vi "CalculateStartupRMS.vi"(8 "error in (no error)":errorcluster, 9 "frequency":dbl, 10 "Motor":T1, 11 "current waveforms":waveform(dbl)[](array[waveform])) -> (0 "error out":errorcluster, 3 "Percent Full Load Amps [%FLA]":dbl)   [LabVIEW 2017, in "McsaAnalysisFunctions.lvlib"]
uses:
  <vilib>/addons/InsightCM/Utilities/Analysis/MCSA/McsaAnalysisFunctions.lvlib
  <vilib>/addons/InsightCM/Utilities/Analysis/MCSA/controls/McsaMotor.ctl
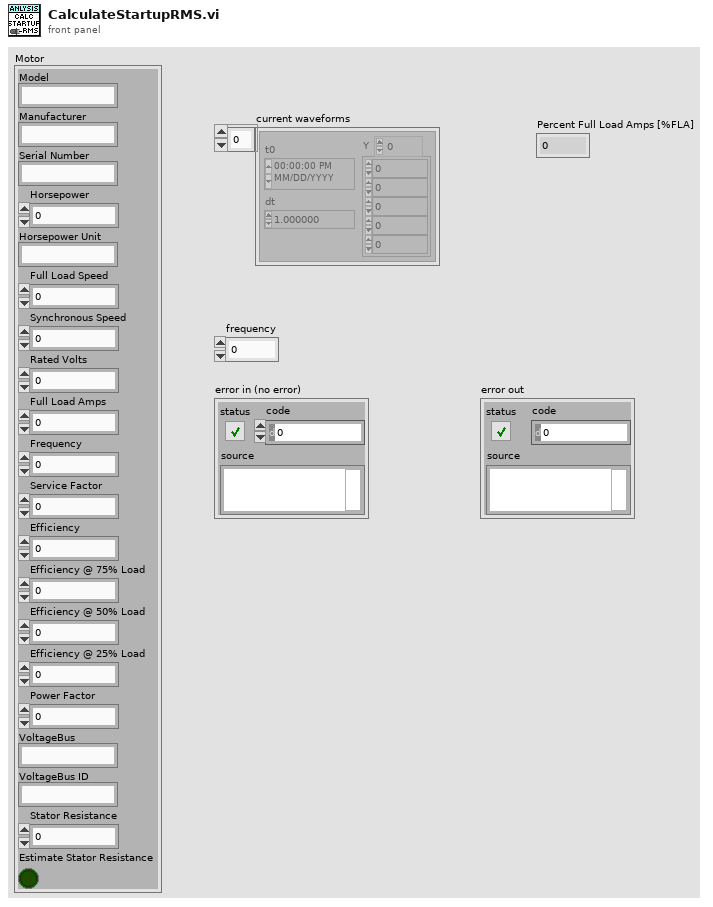
[diagram p1: front panel]
types:
  T1 = typedef "McsaAnalysisFunctions.lvlib/McsaMotor.ctl" = cluster{"Model":string, "Manufacturer":string, "Serial Number":string, "Horsepower":dbl, "Horsepower Unit":string, "Full Load Speed":dbl, "Synchronous Speed":dbl, "Rated Volts":dbl, "Full Load Amps":dbl, "Frequency":dbl, "Service Factor":dbl, "Efficiency":dbl, "Efficiency @ 75% Load":dbl, "Efficiency @ 50% Load":dbl, "Efficiency @ 25% Load":dbl, "Power Factor":dbl, "VoltageBus":string, "VoltageBus ID":string, "Stator Resistance":dbl, "Estimate Stator Resistance":bool}
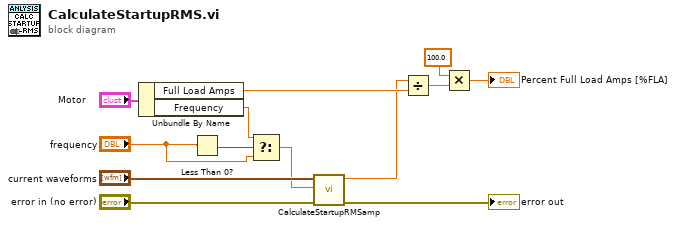
[diagram p0: block diagram]
diagram:
  n1 = Unbundle By Name("Motor") -> ("Full Load Amps"=w10:dbl, "Frequency"=w2:dbl)
  n2 = Less Than 0?(x="frequency") -> (x < 0?=w5:bool)
  n3 = Select(t=w2, s=w5, f="frequency") -> (s? t:f=w4:dbl)
  n4 = call <vilib>:"CalculateStartupRMSamp.vi"("error in (no error)"="error in (no error)", "frequency"=w4, "current waveforms"="current waveforms") -> ("error out"=→"error out":errorcluster, "3-phase Max Startup RMS (rms)"=w6:sgl)  [unwired: 7 in]
  n5 = Divide(x=w6, y=w10) -> (x/y=w11:dbl)
  n6 = Multiply(x=100.0, y=w11) -> (x*y=→"Percent Full Load Amps [%FLA]":dbl)
